vi "Dinamic_function.vi"(9 "balls":T1[](array[typedef]), 10 "IA State":T7={"our_robots"=[], "enemy_robots"=[], "balls"=[], "geometry"={"field_length"=0, "field_width"=0, "goal_width"=0, "goal_depth"=0, "center_circle_radius"=0, "defense_width"=0, "defense_depth"=0, "free_kick_from_defense_dist"=0, "penalty_spot_from_field_line_dist"=0, "penalty_line_from_spot_dist"=0, "half_moon_depth"=0, "half_moon_width"=0}, "IA Judge"={"stage"="", "command"="", "our_goalie_id"=0.0, "enemy_goalie_id"=0.0, "command enum"=enum."Halt", "Time"=enum."Azul"}, "Received Timestamp"=timestamp(0 s since 1904-01-01), "Events"={"Touch"=FALSE, "id touch"=0.0, "Ball out of \nVision"=FALSE, "Ball inside \nGoalie area"=FALSE, "Robot not responding"=FALSE, "Robots responding status"=[1.0, 1.0, 1.0, 1.0, 1.0, 1.0], "Enemy Ball \nPossession"=FALSE, "Id ini Possession"=0.0, "Ball Possesion"=FALSE, "Id Possesion"=0.0, "Ball at\nour goal side"=FALSE, "Ball at\ntouchline"=FALSE, "Ball at\nenemy goal side"=FALSE}}, 11 "Robot in":T2) -> (3 "Numeric":i32)   [LabVIEW 2018]
uses:
  Core/AI Input.ctl
  Core/AI Robot.ctl
  Functions Enum.ctl
  AttackerStates.ctl
  Path Planning/RRT/PathDests.ctl
  Path Planning/RRT/PathDest.ctl
  Core/AI Ball.ctl
  Core/Field Size.ctl
  Core/AI Judge.ctl
  Command Enum.ctl
  Util/Events/Events.ctl
  <vilib>/Analysis/_algsub.llb/Real Vector Norm.vi
  <vilib>/Analysis/NI_AALPro.lvlib
panel:
  out "id 2":u32
  out "id":u32
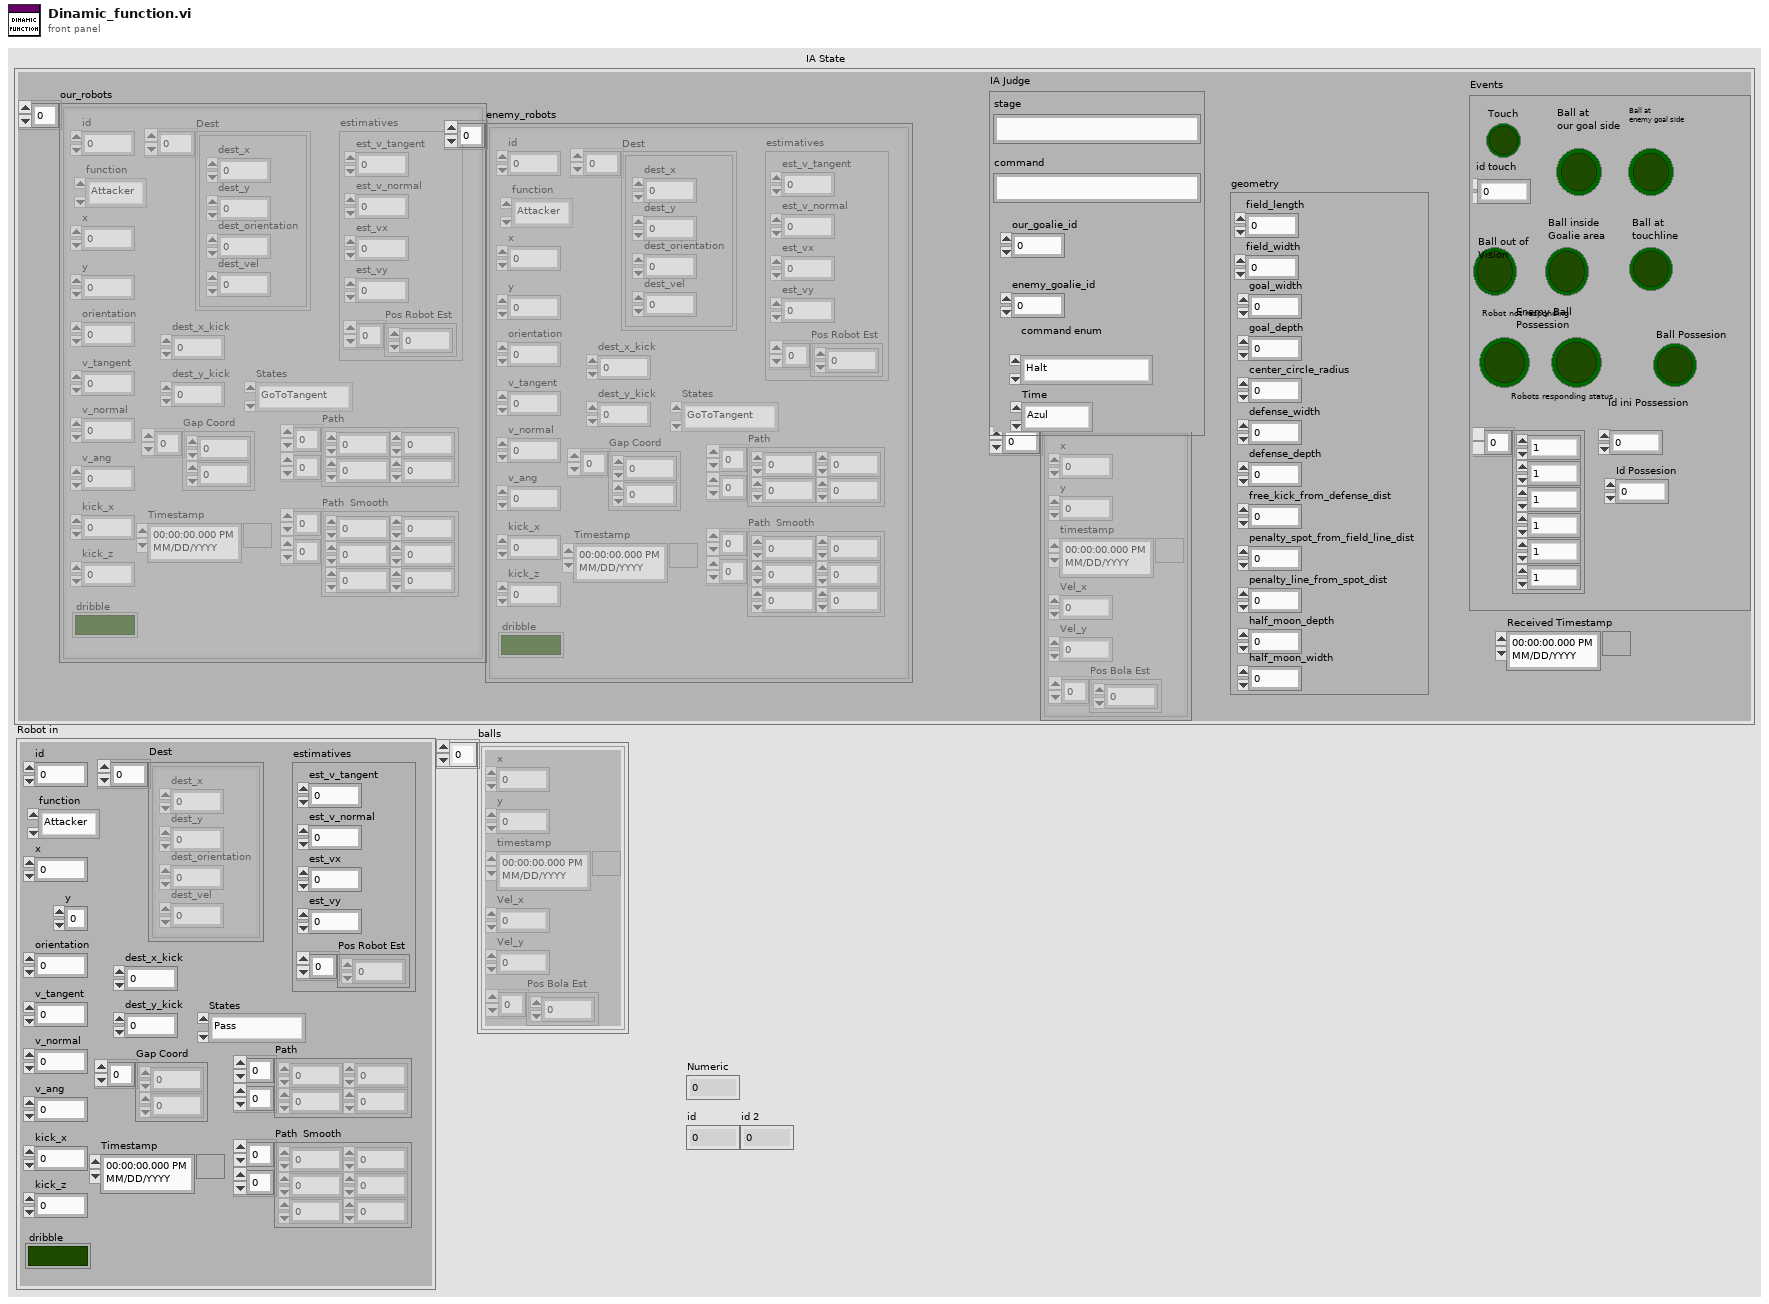
[diagram p1: front panel]
types:
  T1 = typedef "AI Ball.ctl" = cluster{"x":dbl, "y":dbl, "timestamp":timestamp, "Vel_x":dbl, "Vel_y":dbl, "Pos Bola Est":dbl[]}
  T2 = typedef "AI Robot.ctl" = cluster{"id":u32, "function":T3, "x":dbl, "y":dbl, "orientation":dbl, "v_tangent":dbl, "v_normal":dbl, "v_ang":dbl, "kick_x":dbl, "kick_z":dbl, "dribble":bool, "Timestamp":timestamp, "estimatives":cluster{"est_v_tangent":dbl, "est_v_normal":dbl, "est_vx":dbl, "est_vy":dbl, "Pos Robot Est":dbl[]}, "dest_x_kick":dbl, "dest_y_kick":dbl, "Gap Coord":dbl[], "States":T4, "Path ":dbl[][], "Path  Smooth":dbl[][], "Dest":T5}
  T3 = typedef "Functions Enum.ctl" = enum16{"Attacker", "Goalie", "Defender", "Striker", "Goto 0", "Dummy", "Kicker", "ZigZag"}
  T4 = typedef "AttackerStates.ctl" = enum16{"Pass", "GoToTangent", "BallGetting", "GoToKick", "Rotate anti-clockwise", "Rotate Clockwise", ""}
  T5 = typedef "PathDests.ctl" = T6[]
  T6 = typedef "PathDest.ctl" = cluster{"dest_x":dbl, "dest_y":dbl, "dest_orientation":dbl, "dest_vel":dbl}
  T7 = typedef "AI Input.ctl" = cluster{"our_robots":T2[], "enemy_robots":T2[], "balls":T1[], "geometry":T8, "IA Judge":T9, "Received Timestamp":timestamp, "Events":T11}
  T8 = typedef "Field Size.ctl" = cluster{"field_length":u32, "field_width":u32, "goal_width":u32, "goal_depth":u32, "center_circle_radius":u32, "defense_width":u32, "defense_depth":u32, "free_kick_from_defense_dist":u32, "penalty_spot_from_field_line_dist":u32, "penalty_line_from_spot_dist":u32, "half_moon_depth":u32, "half_moon_width":u32}
  T9 = typedef "AI Judge.ctl" = cluster{"stage":string, "command":string, "our_goalie_id":dbl, "enemy_goalie_id":dbl, "command enum":T10, "Time":enum16{"Azul", "Amarelo"}}
  T10 = typedef "Command Enum.ctl" = enum16{"Halt", "Stop", "Force Start", "PKA Normal Start", "Prepare Kickoff Ally", "PKE Normal Start", "Prepare Kickoff Enemy", "Prepare Penalty Ally", "PPA Normal Start", "Prepare Penalty Enemy", "PPE Normal Start", "Ball Placement Enemy Up", "Ball Placement Enemy Down", "Ball Placement Ally Up", "Ball Placement Ally Mid", "Ball Placement Ally Down", "Indirect Free Enemy", "Indirect Free Ally", "Timeout Enemy", "Timeout Ally", "Goal Enemy", "Goal Ally", "Normal Half Time", "Extra Time Break", "Extra Half Time", "None", "Post Game"}
  T11 = typedef "Events.ctl" = cluster{"Touch":bool, "id touch":dbl, "Ball out of \nVision":bool, "Ball inside \nGoalie area":bool, "Robot not responding":bool, "Robots responding status":dbl[], "Enemy Ball \nPossession":bool, "Id ini Possession":dbl, "Ball Possesion":bool, "Id Possesion":dbl, "Ball at\nour goal side":bool, "Ball at\ntouchline":bool, "Ball at\nenemy goal side":bool}
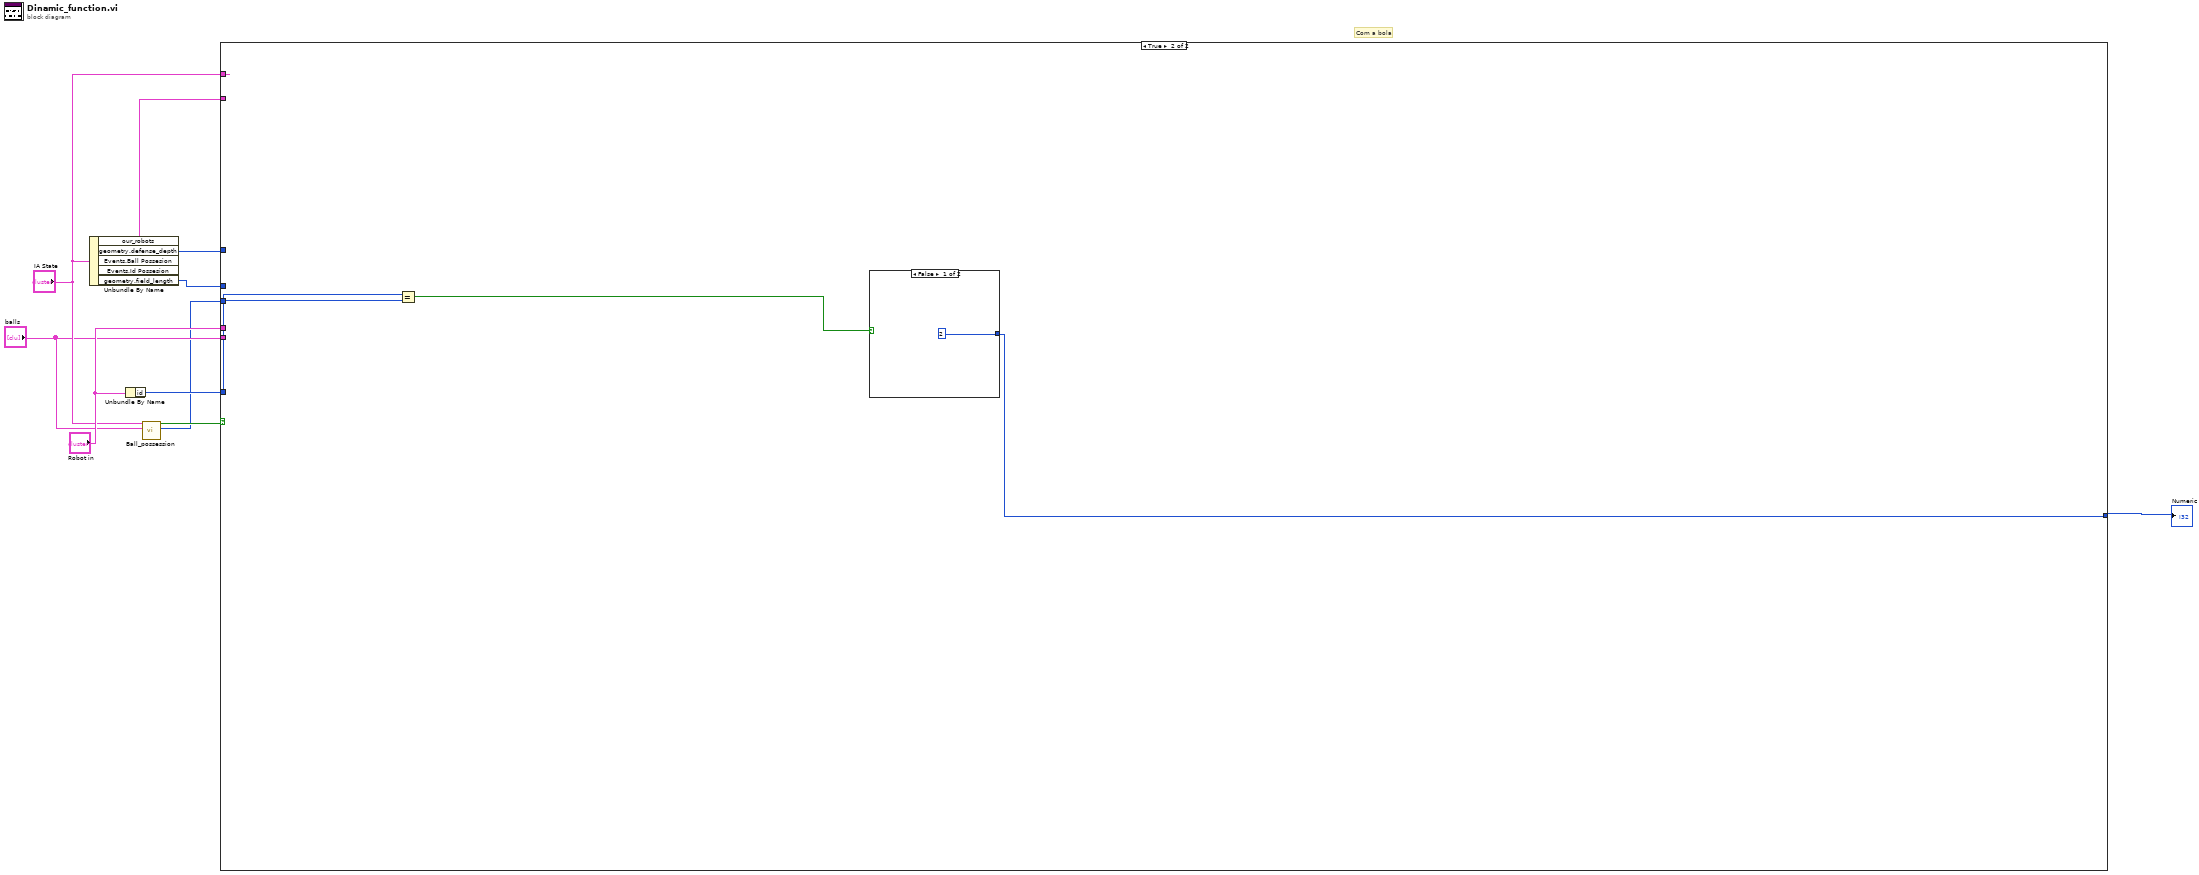
[diagram p0: block diagram]
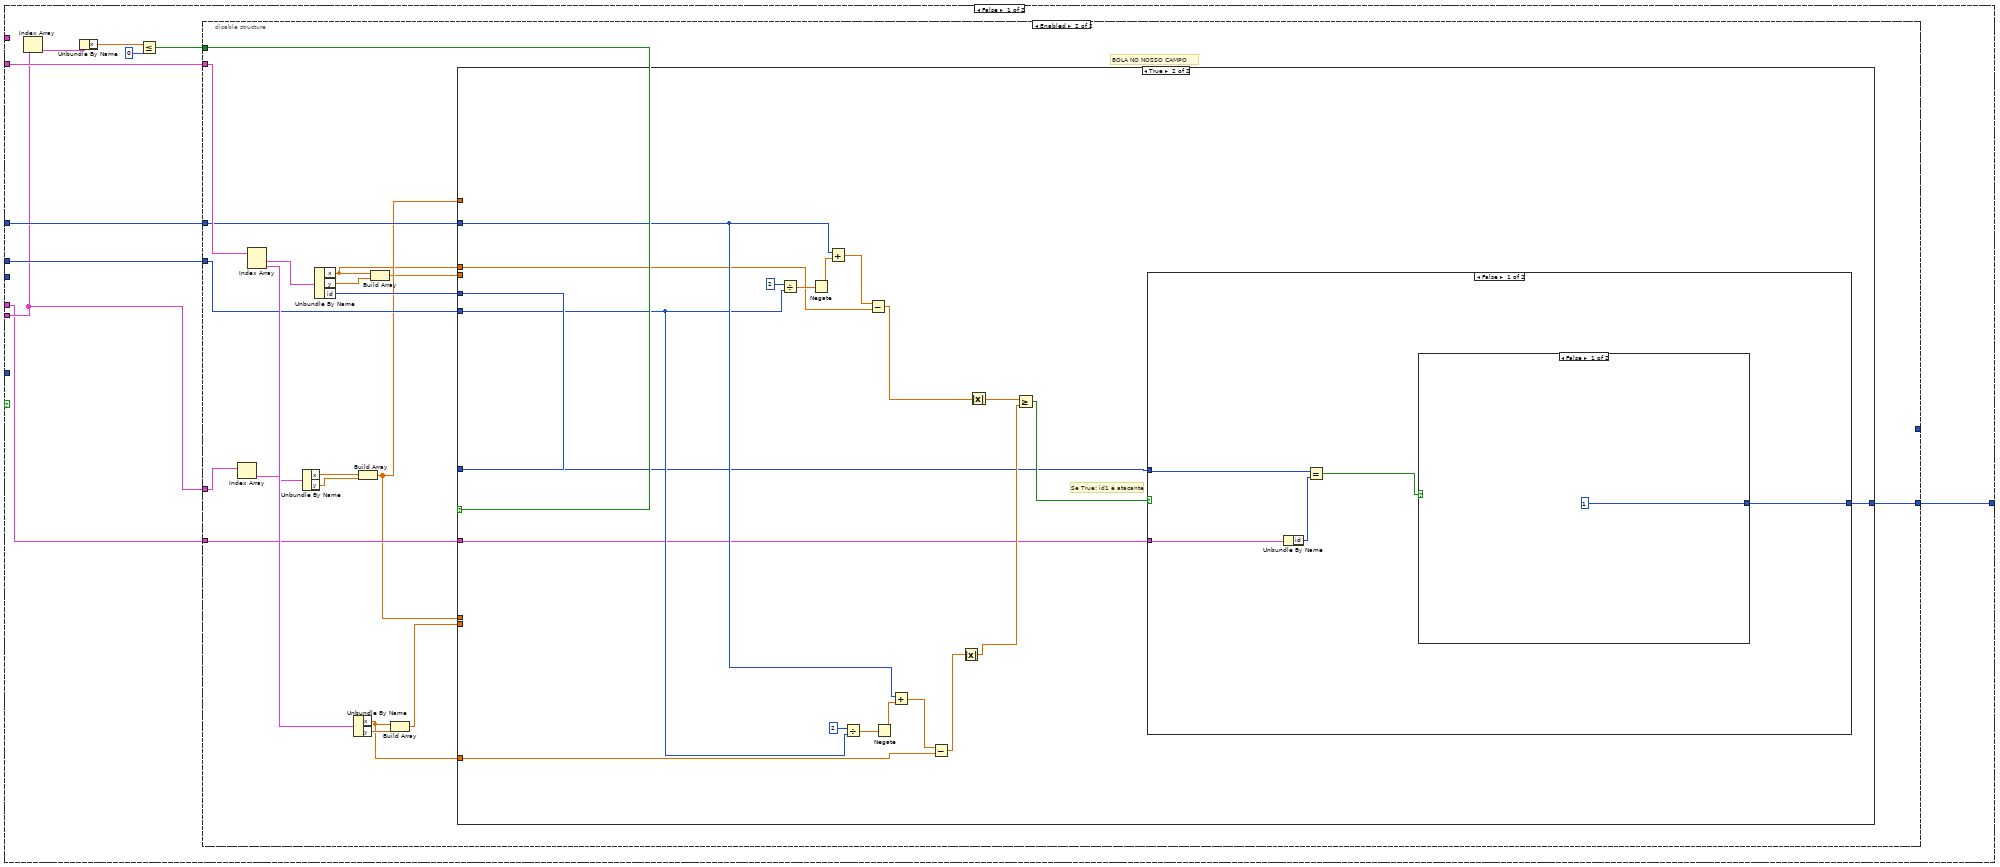
[diagram p2: hidden frame]
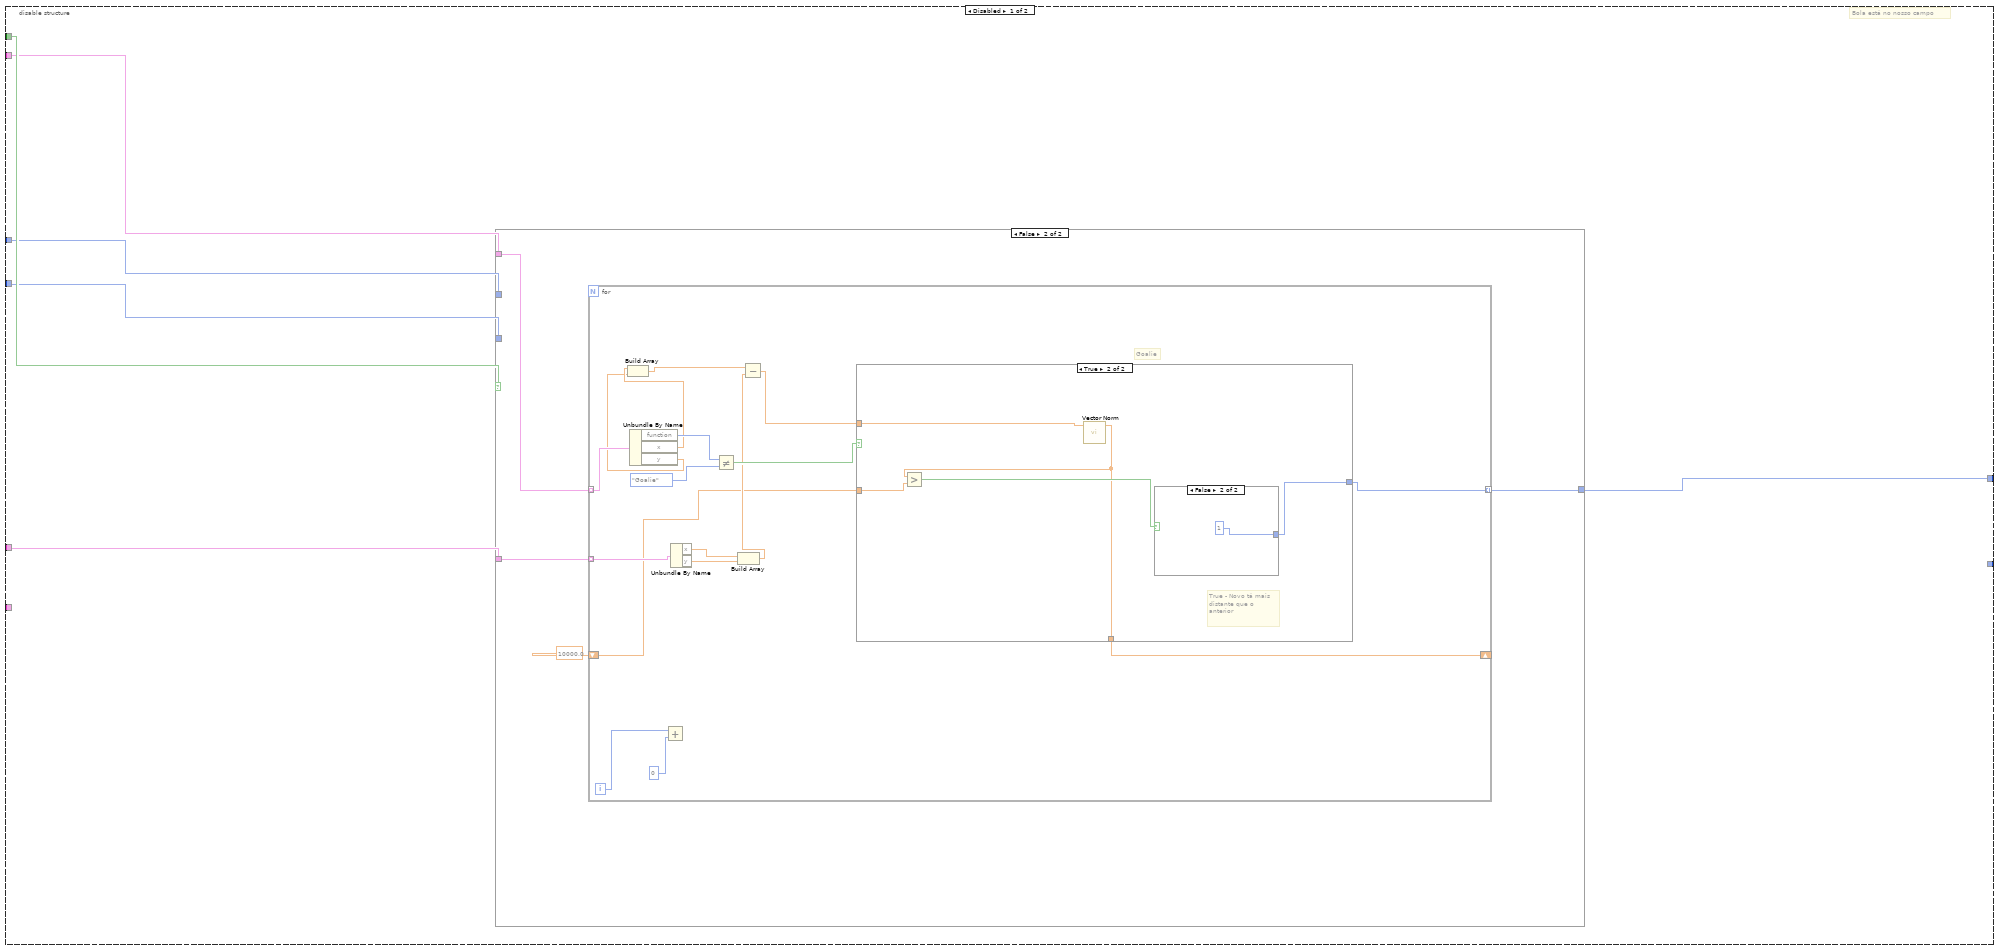
[diagram p3: hidden frame]
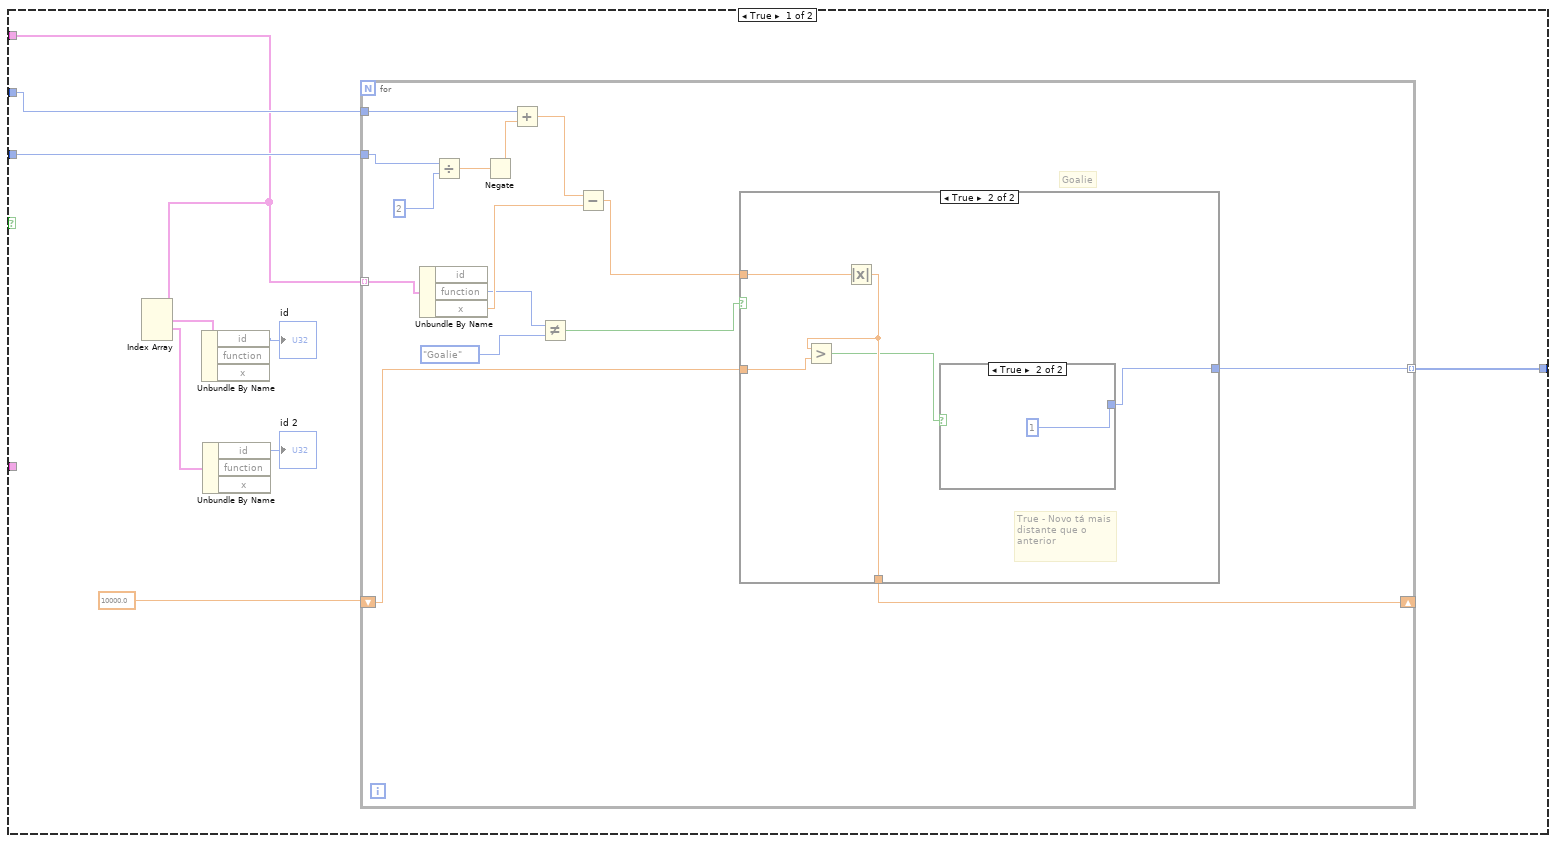
[diagram p4: hidden frame]
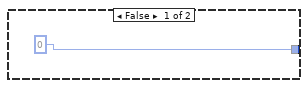
[diagram p5: hidden frame]
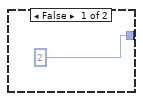
[diagram p6: hidden frame]
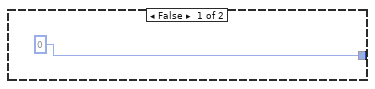
[diagram p7: hidden frame]
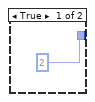
[diagram p8: hidden frame]
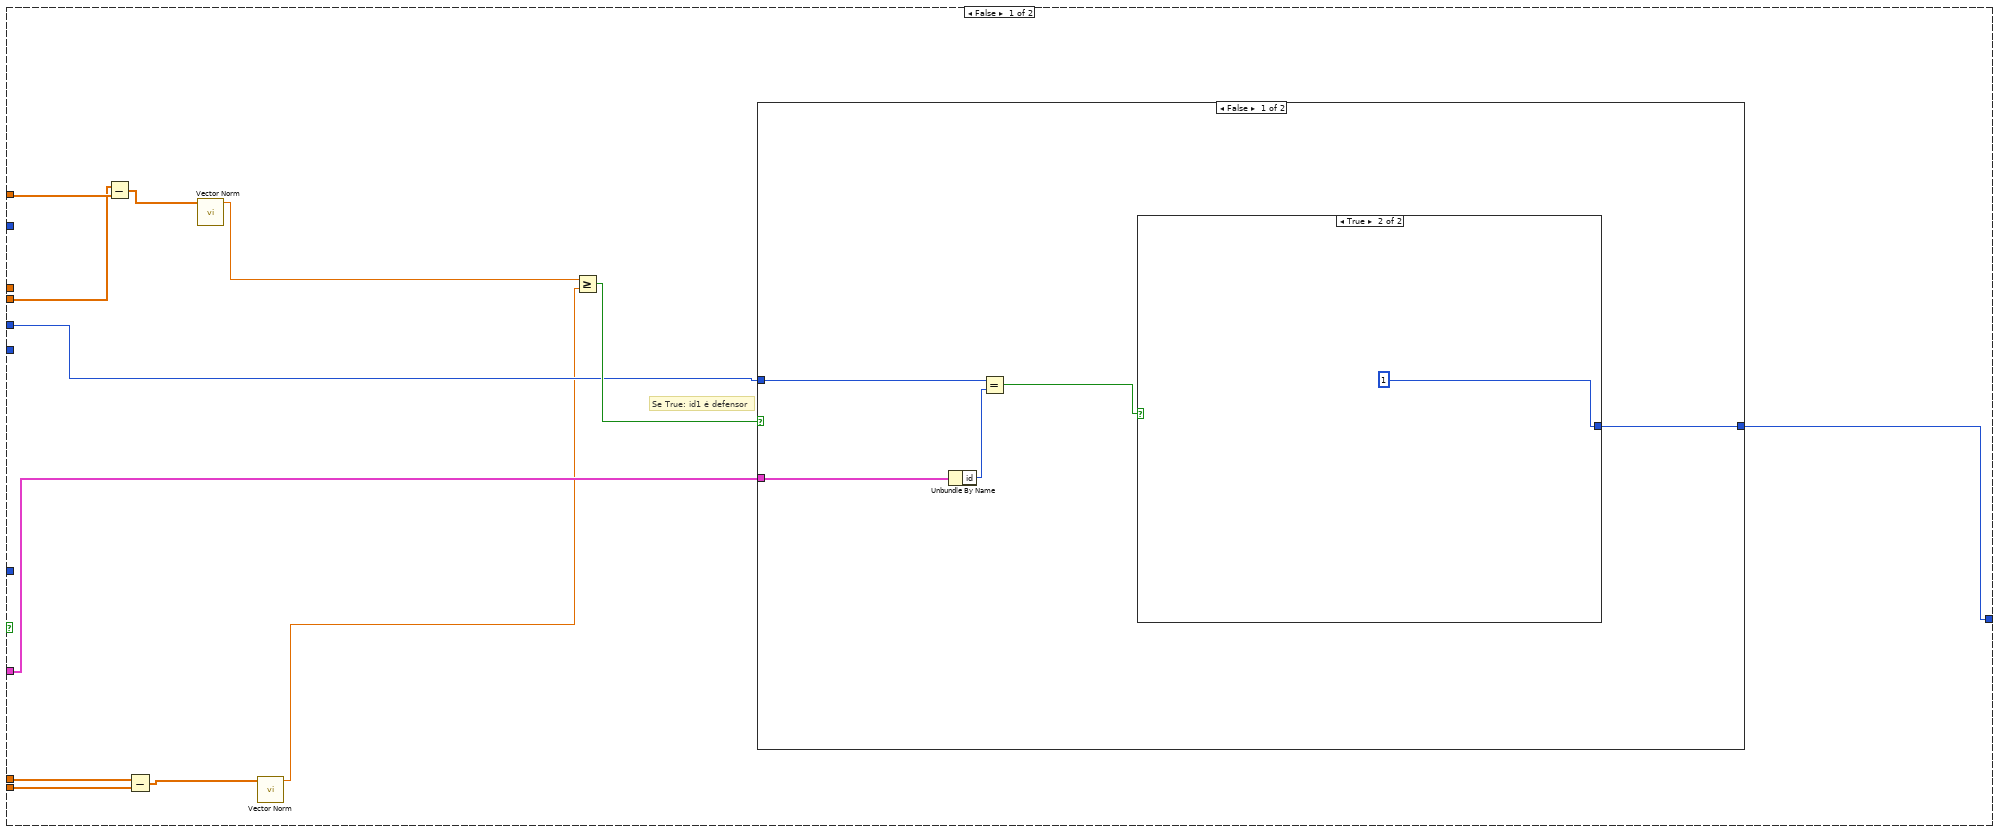
[diagram p9: hidden frame]
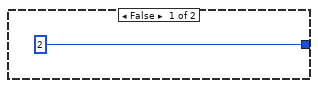
[diagram p10: hidden frame]
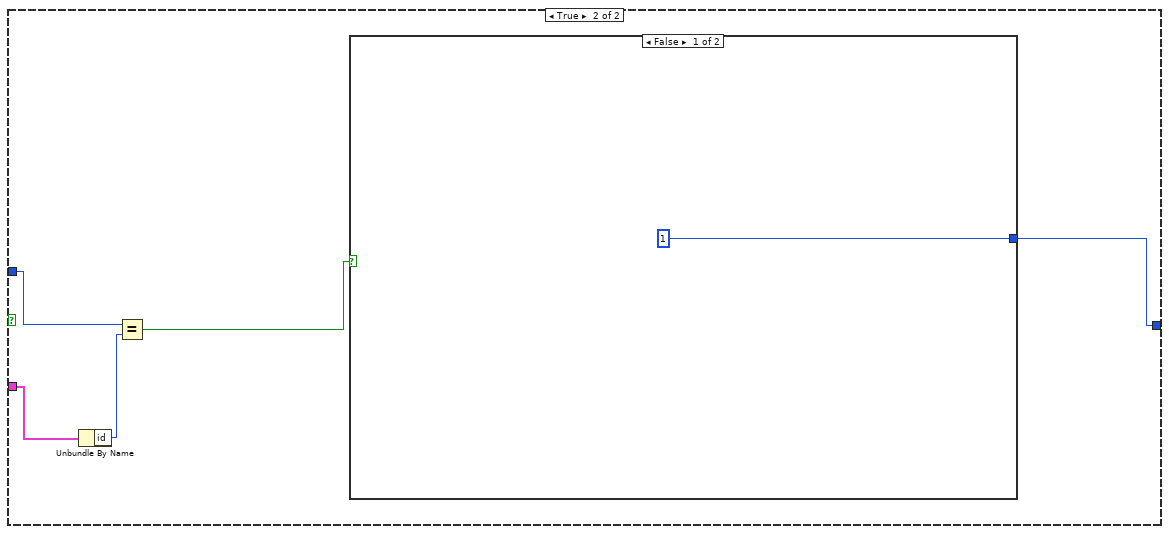
[diagram p11: hidden frame]
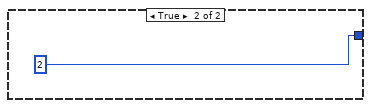
[diagram p12: hidden frame]
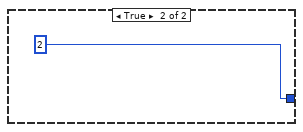
[diagram p13: hidden frame]
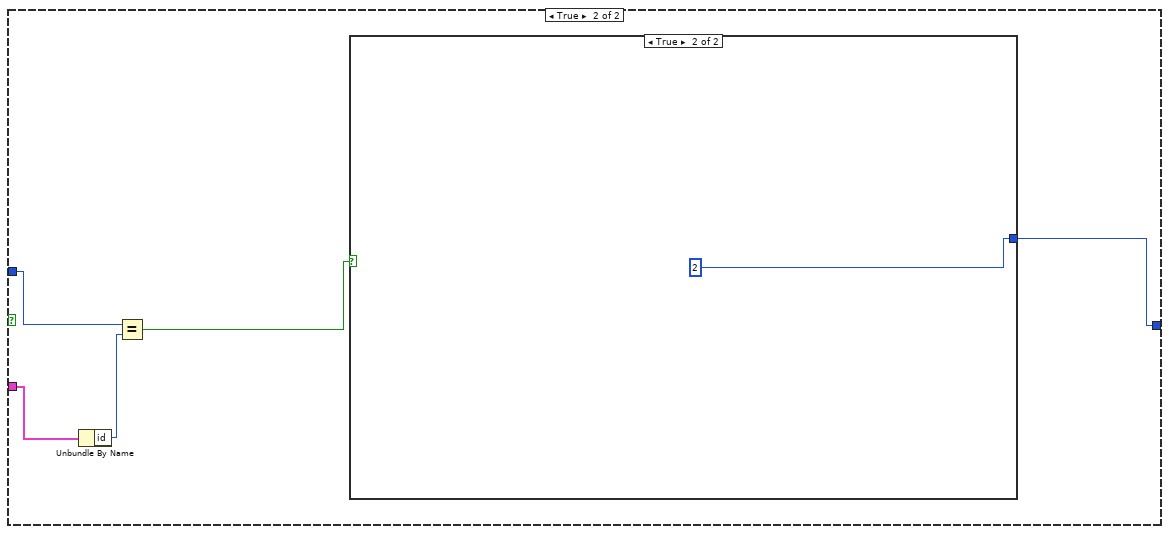
[diagram p14: hidden frame]
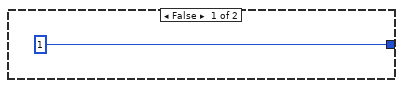
[diagram p15: hidden frame]
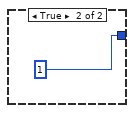
[diagram p16: hidden frame]
diagram:
  # "Com a bola"
  n1 = Unbundle By Name("IA State") -> ("our_robots"=w7:T2[], "geometry.defense_depth"=w8:u32, "geometry.field_length"=w6:u32)  [unwired: 2 out]
  n2 = Unbundle By Name("Robot in") -> ("id"=w10:u32)
  n3 = call "Ball_possession.vi"("balls"="balls", "IA State"="IA State") -> ("id"=w1:u32, "Boolean"=w2:bool)  [unwired: 8 in]
  n4 = case shown="True" w2 {
    tunnel: w1 -> [_ w171]
    tunnel: w10 -> [_ w170]
    tunnel: "Robot in" -> [w12 _]
    tunnel: "IA State" -> [_ _]
    tunnel: "balls" -> [w13 _]
    tunnel: w8 -> [w17 _]
    tunnel: w7 -> [w16 _]
    tunnel: w6 -> [w14 _]
    tunnel: [w11 w168] -> w5
    frame False {
      n5 = Index Array(array=w13) -> (element=w15:T1)  [unwired: 1 in]
      n6 = Unbundle By Name(w15) -> ("x"=w20:dbl)
      n7 = Less Or Equal?(x=w20, y=0) -> (x <= y?=w18:bool)
      n8 = disable-structure shown="Enabled" {
        disable-tunnel: w18 -> [w26 w107]
        disable-tunnel: w17 -> [w25 w102]
        disable-tunnel: w16 -> [w24 w104]
        disable-tunnel: w14 -> [w23 w103]
        disable-tunnel: w13 -> [w22 w96]
        disable-tunnel: [w21 _] -> _
        disable-tunnel: w12 -> [_ w101]
        disable-tunnel: [_ w100] -> w11
        frame Disabled {
          # "Bola está no nosso campo"
          n9 = case shown="False" w26 {
            tunnel: w25 -> [w34 _]
            tunnel: w24 -> [w31 w62]
            tunnel: w23 -> [w35 _]
            tunnel: [w32 w61] -> w21
            tunnel: w22 -> [_ w60]
            frame True {
              n10 = Index Array(array=w31) -> (element #1=w30:T2, element #2=w29:T2)  [unwired: 3 in, 1 out]
              n11 = Unbundle By Name(w30) -> ("id"=→"id":u32)  [unwired: 2 out]
              n12 = Unbundle By Name(w29) -> ("id"=→"id 2":u32)  [unwired: 2 out]
              n13 = for {
                shift-right: [w39] -> _
                shift-left: 10000.0 -> [w36]
                tunnel: w35 -> [w50]
                tunnel: w34 -> [w47]
                tunnel: [w38] -> w32 mode=indexing
                tunnel: w31 -> [w37] mode=indexing
                # "Goalie"
                n14 = Unbundle By Name(w37) -> ("function"=w42:T3, "x"=w44:dbl)  [unwired: 1 out]
                n15 = Divide(x=w50, y=2) -> (x/y=w48:dbl)
                n16 = Negate(x=w48) -> (-x=w46:dbl)
                n17 = Add(x=w47, y=w46) -> (x+y=w45:dbl)
                n18 = Not Equal?(x=w42, y=enum16{"Goalie", ""}."Goalie") -> (x != y?=w41:bool)
                n19 = Subtract(x=w45, y=w44) -> (x-y=w40:dbl)
                n20 = case shown="True" w41 {
                  tunnel: w40 -> [_ w56]
                  tunnel: [_ w55] -> w39
                  tunnel: w36 -> [_ w54]
                  tunnel: [0 w52] -> w38
                  frame False {
                  }
                  frame True {
                    # "True - Novo tá mais distante que o anterior"
                    n21 = Absolute Value(x=w56) -> (abs(x)=w55:dbl)
                    n22 = Greater?(x=w55, y=w54) -> (0:w53:bool)
                    n23 = case shown="True" w53 {
                      tunnel: [2 1] -> w52
                      frame False {
                      }
                      frame True {
                      }
                    }
                  }
                }
              }
            }
            frame False {
              n24 = for {
                tunnel: w62 -> [w79] mode=indexing
                shift-right: [w74] -> _
                shift-left: 10000.0 -> [w65]
                tunnel: [w67] -> w61 mode=indexing
                tunnel: w60 -> [w66] mode=indexing
                i -> [w64]
                # "Goalie"
                n25 = Unbundle By Name(w79) -> ("function"=w77:T3, "x"=w71:dbl, "y"=w70:dbl)
                n26 = Build Array(w71, w70) -> (w69:dbl[])
                n27 = Add(x=w64, y=0) -> ()  [unwired: 1 out]
                n28 = Unbundle By Name(w66) -> ("x"=w73:dbl, "y"=w72:dbl)
                n29 = Not Equal?(x=w77, y=enum16{"Goalie", ""}."Goalie") -> (x != y?=w76:bool)
                n30 = Build Array(w73, w72) -> (w68:dbl[])
                n31 = Subtract(x=w69, y=w68) -> (x-y=w75:dbl[])
                n32 = case shown="True" w76 {
                  tunnel: w75 -> [_ w83]
                  tunnel: [_ w82] -> w74
                  tunnel: w65 -> [_ w85]
                  tunnel: [0 w81] -> w67
                  frame False {
                  }
                  frame True {
                    # "True - Novo tá mais distante que o anterior"
                    n33 = call-poly <vilib>:"Vector Norm.vi"("Input Vector"=w83) -> ("norm"=w82:dbl)  [unwired: 9 in, 1 out]
                    n34 = Greater?(x=w82, y=w85) -> (0:w84:bool)
                    n35 = case shown="False" w84 {
                      tunnel: [2 1] -> w81
                      frame True {
                      }
                      frame False {
                      }
                    }
                  }
                }
              }
            }
          }
        }
        frame Enabled {
          # "BOLA NO NOSSO CAMPO"
          n36 = Index Array(array=w96) -> (element=w95:T1)  [unwired: 1 in]
          n37 = Index Array(array=w104) -> (element #1=w106:T2, element #2=w105:T2)  [unwired: 2 in]
          n38 = Unbundle By Name(w95) -> ("x"=w94:dbl, "y"=w93:dbl)
          n39 = Unbundle By Name(w106) -> ("x"=w89:dbl, "y"=w97:dbl, "id"=w99:u32)
          n40 = Unbundle By Name(w105) -> ("x"=w88:dbl, "y"=w98:dbl)
          n41 = Build Array(w94, w93) -> (w91:dbl[])
          n42 = Build Array(w89, w97) -> (w90:dbl[])
          n43 = Build Array(w88, w98) -> (w92:dbl[])
          n44 = case shown="True" w107 {
            tunnel: w103 -> [_ w144]
            tunnel: w102 -> [_ w145]
            tunnel: w101 -> [w118 w138]
            tunnel: w99 -> [_ w137]
            tunnel: [w108 w136] -> w100
            tunnel: w99 -> [w117 _]
            tunnel: w91 -> [w116 _]
            tunnel: w92 -> [w115 _]
            tunnel: w91 -> [w114 _]
            tunnel: w90 -> [w113 _]
            tunnel: w89 -> [_ w135]
            tunnel: w88 -> [_ w134]
            frame False {
              # "Se True: id1 é defensor"
              n45 = Subtract(x=w113, y=w114) -> (x-y=w112:dbl[])
              n46 = Subtract(x=w116, y=w115) -> (x-y=w110:dbl[])
              n47 = call-poly <vilib>:"Vector Norm.vi"("Input Vector"=w112) -> ("norm"=w111:dbl)  [unwired: 9 in, 1 out]
              n48 = call-poly <vilib>:"Vector Norm.vi"("Input Vector"=w110) -> ("norm"=w109:dbl)  [unwired: 9 in, 1 out]
              n49 = Greater Or Equal?(x=w111, y=w109) -> (x >= y?=w119:bool)
              n50 = case shown="False" w119 {
                tunnel: w118 -> [w122 w131]
                tunnel: w117 -> [w123 w130]
                tunnel: [w120 w127] -> w108
                frame False {
                  n51 = Unbundle By Name(w122) -> ("id"=w124:u32)
                  n52 = Equal?(x=w123, y=w124) -> (x = y?=w121:bool)
                  n53 = case shown="True" w121 {
                    tunnel: [2 1] -> w120
                    frame False {
                    }
                    frame True {
                    }
                  }
                }
                frame True {
                  n54 = Unbundle By Name(w131) -> ("id"=w129:u32)
                  n55 = Equal?(x=w130, y=w129) -> (x = y?=w128:bool)
                  n56 = case shown="False" w128 {
                    tunnel: [1 2] -> w127
                    frame False {
                    }
                    frame True {
                    }
                  }
                }
              }
            }
            frame True {
              # "Se True: id1 é atacante"
              n57 = Divide(x=u32 2, y=w144) -> (x/y=w153:dbl)
              n58 = Negate(x=w153) -> (-x=w152:dbl)
              n59 = Add(x=w145, y=w152) -> (x+y=w151:dbl)
              n60 = Divide(x=u32 2, y=w144) -> (x/y=w149:dbl)
              n61 = Subtract(x=w151, y=w135) -> (x-y=w143:dbl)
              n62 = Negate(x=w149) -> (-x=w148:dbl)
              n63 = Add(x=w145, y=w148) -> (x+y=w147:dbl)
              n64 = Subtract(x=w147, y=w134) -> (x-y=w142:dbl)
              n65 = Absolute Value(x=w142) -> (abs(x)=w140:dbl)
              n66 = Absolute Value(x=w143) -> (abs(x)=w141:dbl)
              n67 = Greater Or Equal?(x=w141, y=w140) -> (x >= y?=w139:bool)
              n68 = case shown="False" w139 {
                tunnel: w138 -> [w156 w165]
                tunnel: w137 -> [w157 w164]
                tunnel: [w154 w161] -> w136
                frame False {
                  n69 = Unbundle By Name(w156) -> ("id"=w158:u32)
                  n70 = Equal?(x=w157, y=w158) -> (x = y?=w155:bool)
                  n71 = case shown="False" w155 {
                    tunnel: [1 2] -> w154
                    frame False {
                    }
                    frame True {
                    }
                  }
                }
                frame True {
                  n72 = Unbundle By Name(w165) -> ("id"=w163:u32)
                  n73 = Equal?(x=w164, y=w163) -> (x = y?=w162:bool)
                  n74 = case shown="True" w162 {
                    tunnel: [1 2] -> w161
                    frame False {
                    }
                    frame True {
                    }
                  }
                }
              }
            }
          }
        }
      }
    }
    frame True {
      n75 = Equal?(x=w171, y=w170) -> (x = y?=w169:bool)
      n76 = case shown="False" w169 {
        tunnel: [2 1] -> w168
        frame False {
        }
        frame True {
        }
      }
    }
  }
  "Numeric" <- w5
